vi "Get Image Grab State.vi"(8 "error in (no error)":errorcluster, 11 "cam cal status":string) -> (0 "error out":errorcluster, 3 "notification":string)   [LabVIEW 2020]
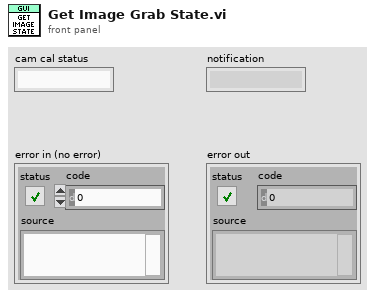
[diagram p1: front panel]
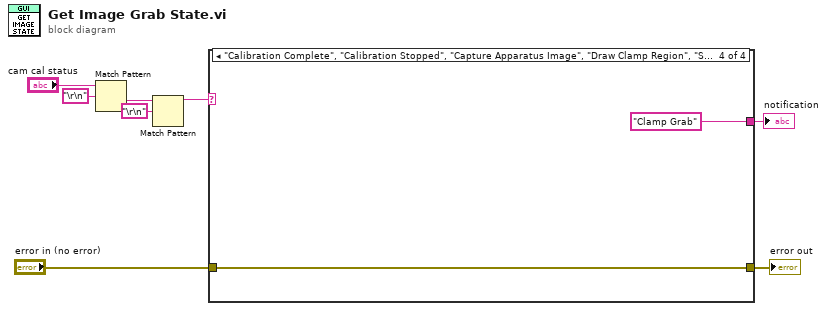
[diagram p0: block diagram]
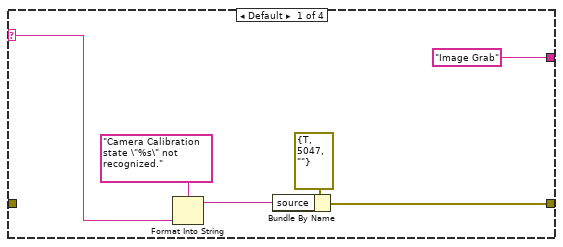
[diagram p2: hidden frame]
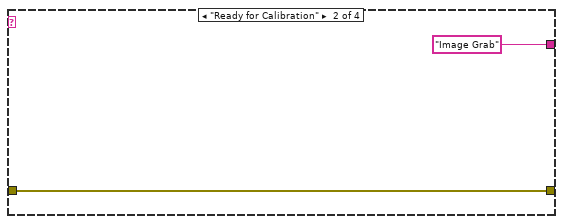
[diagram p3: hidden frame]
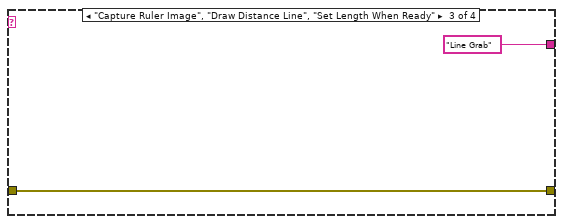
[diagram p4: hidden frame]
diagram:
  n1 = Match Pattern(string="cam cal status", regular expression="\r\n") -> (after substring=w3:string)  [unwired: 1 in, 3 out]
  n2 = Match Pattern(string=w3, regular expression="\r\n") -> (before substring=w2:string)  [unwired: 1 in, 3 out]
  n3 = case shown="\"Calibration Complete\", \"Calibration Stopped\", \"Capture Apparatus Image\", \"Draw Clamp Region\", \"Set Clamp When Ready\", \"Test and Save\"" w2 {
    selector: w2 -> [w11 _ _ _]
    tunnel: "error in (no error)" -> [_ w15 w18 w19]
    tunnel: [w13 w15 w18 w19] -> w8
    tunnel: ["Image Grab" ("notification") "Image Grab" ("notification") "Line Grab" ("notification") "Clamp Grab" ("notification")] -> w1
    frame Default {
      n4 = Format Into String(format string="Camera Calibration state \"%s\" not recognized.", w11) -> (resulting string=w10:string)  [unwired: 2 in, 1 out]
      n5 = Bundle By Name(cluster=errorcluster {"status"=TRUE, "code"=5047, "source"=""} ("error in (no error)"), "source"=w10) -> (w13:errorcluster)
    }
    frame "Ready for Calibration" {
    }
    frame "Capture Ruler Image", "Draw Distance Line", "Set Length When Ready" {
    }
    frame "Calibration Complete", "Calibration Stopped", "Capture Apparatus Image", "Draw Clamp Region", "Set Clamp When Ready", "Test and Save" {
    }
  }
  "error out" <- w8
  "notification" <- w1
